vi "Start_Stop AQ.vi"(8 "error in (no error)":errorcluster, 10 "Start_Stop":bool, 11 "Acquisition in":refnum<class "Acquisition.lvclass">) -> (0 "error out":errorcluster, 3 "Acquisition out":refnum<class "Acquisition.lvclass">)   [LabVIEW 2020, in "Acquisition.lvlib" / "Acquisition.lvclass"]
uses:
  Acquisition.lvclass
  Acquisition.lvclass/Acquisition.ctl
  <vilib>/ActorFramework/Actor/Actor.lvclass
  Businness Logic/Businness Logic Messages/Update Status Msg/Update Status Msg.lvclass
  C:/Program Files (x86)/National Instruments/LabVIEW 2020/vi.lib/ActorFramework/Actor/Actor.lvclass
  D:/Storage/Source Code/Clase AF/ClaseAF/08 Acquisition AF/Acquisition/Acquisition/Acquisition.lvclass
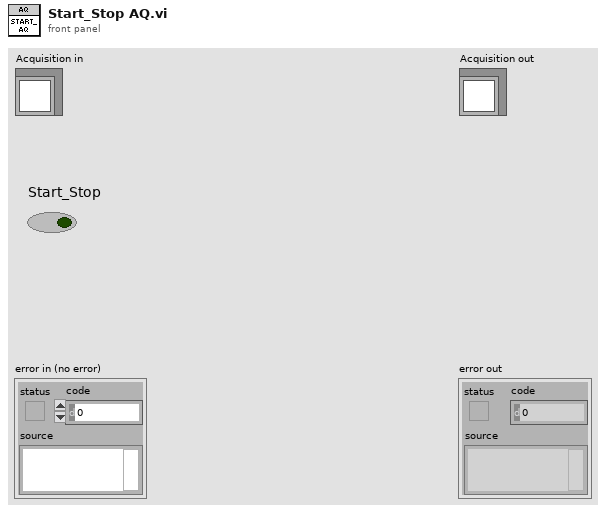
[diagram p1: front panel]
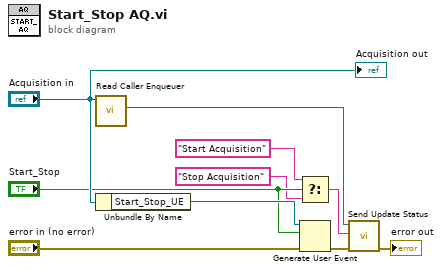
[diagram p0: block diagram]
diagram:
  n1 = call <vilib>:"Read Caller Enqueuer.vi"("Actor"="Acquisition in") -> ("Caller Enqueuer"=w7:refnum<class "Message Enqueuer.lvclass">)  [unwired: 10 in]
  n2 = Unbundle By Name("Acquisition in") -> ("Start_Stop_UE"=w9:refnum<user-event>)
  n3 = Select(t="Start Acquisition", s="Start_Stop", f="Stop Acquisition") -> (s? t:f=w5:string)
  n4 = Generate User Event(user event=w9, event data cluster="Start_Stop", error in="error in (no error)") -> (error out=w2:errorcluster)  [unwired: 1 in, 1 out]
  n5 = call "Send Update Status.vi"("error in (no error)"=w2, "Status"=w5, "Message Enqueuer"=w7) -> ("error out"=→"error out":errorcluster)  [unwired: 7 in, 1 out]
  "Acquisition out" <- "Acquisition in"
